vi "ObjCacher-Viewer.vi"(1 "type":variant, 7 "typeKey(\"\" to use DataTypeDescription)":string, 11 "error in (no error)":errorcluster, 12 "type group(\"\")":string) -> (4 "cacher":variant, 6 "Global Cacher":variant, 15 "error out":errorcluster)   [LabVIEW 2017, in "ObjectCacherAPI.lvlib"]
uses:
  ObjectCacherAPI.lvlib
  a8f93028-50f0-47dd-85bb-77c48d180597.vi
  Data/_support/Get DataType Description String.vi
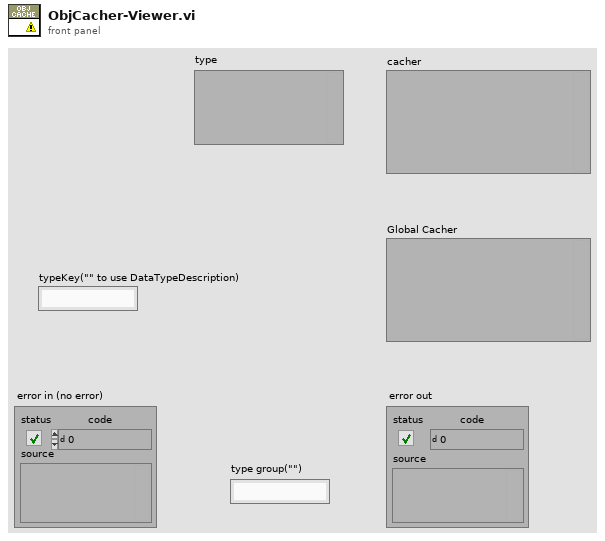
[diagram p1: front panel]
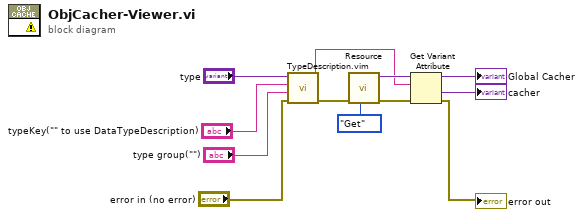
[diagram p0: block diagram]
diagram:
  n1 = call "TypeDescription.vim"("error in"="error in (no error)", "type group(\"\")"="type group(\"\")", "typeKey(\"\" to use DataTypeDescription)"="typeKey(\"\" to use DataTypeDescription)", "type"="type") -> ("error out"=w10:errorcluster, "String"=w1:string)  [unwired: 6 in]
  n2 = call "Resource.vi"("action"=enum16{"Get", "Lock", "unlock"}."Get" ("Set(T)/Get(F)"), "error in (no error)"=w10) -> ("error out"=w9:errorcluster, "GlobalCacher"=w12:variant)  [unwired: 7 in, 1 out]
  n3 = Get Variant Attribute(Variant=w12, name=w1, error in=w9) -> (duplicate Variant=→"Global Cacher":variant, value=→"cacher":variant, error out=→"error out":errorcluster)  [unwired: 1 in, 1 out]
